vi "DataReadTxtGen.vi"(6 "VarParIndex":i32, 8 "error in":errorcluster, 9 "ScanlistIndex":i32, 10 "chemin Data":path, 11 "Chemin Header":path) -> (0 "error out":errorcluster, 1 "Y Array":dbl[](array[numeric]), 2 "X Array":dbl[](array[numeric]), 3 "Data Preview":string[][](array[string]), 4 "CurveName":string, 5 "VarPar":string)   [LabVIEW 2010]
doc: "Ce VI lit les données contenu dans le fichier de sauvegarde automatique. Ces données correspondent aux valeurs prises lors du dernier balayage. La sauvegarde automatique est effectué après chaque acquisition."
uses:
  H:/Mes documents/Programmes Labview/LabScan/LabScanV1A/Interface Class/ScanParams.ctl
  H:/Mes documents/Programmes Labview/LabScan/LabScanV1A/Interface Class/Interface.lvclass
panel:
  out "enregistrement(s)":T1={"Entête"="", "Scan list"=[], "NbCourbe"=1, "IndCourbe"=0, "NomDon"=["RTêta;", "X&Y;"], "Session "=0, "Date"="", "Time"="", "VarParams"=[], "UserName"="", "ScanTableSize"=[]} caption="ScanParams"
  out "AllData":dbl[][](array[numeric]) format="%#.16f"
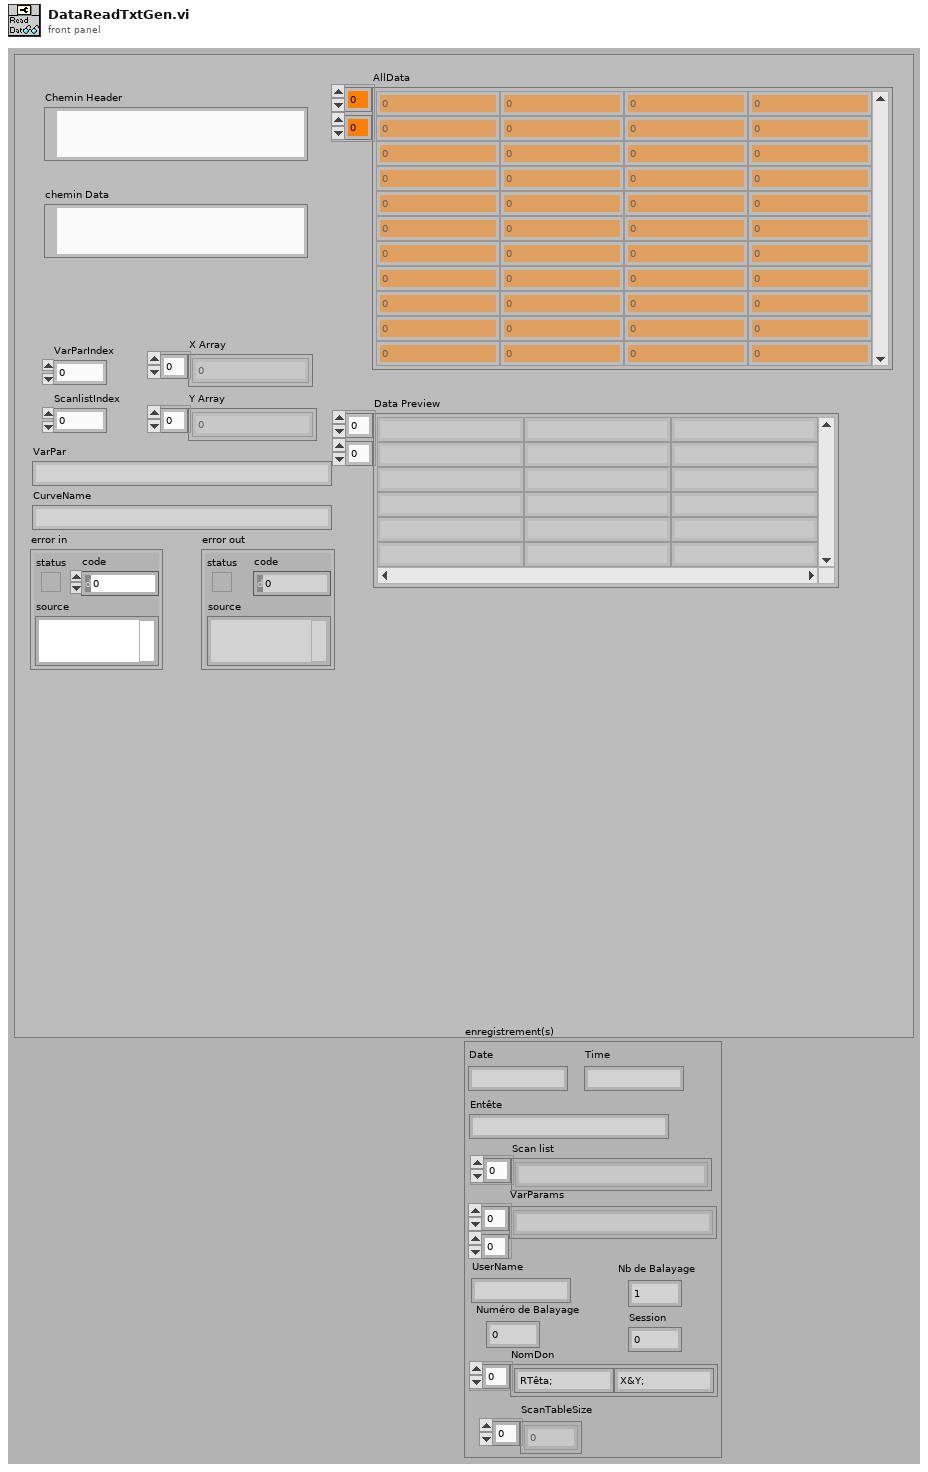
[diagram p1: front panel]
types:
  T1 = typedef "Interface.lvclass/ScanParams.ctl" = cluster{"Entête":string, "Scan list":string[], "NbCourbe":i32, "IndCourbe":i64, "NomDon":string[], "Session ":i32, "Date":string, "Time":string, "VarParams":string[][], "UserName":string, "ScanTableSize":i32[]}
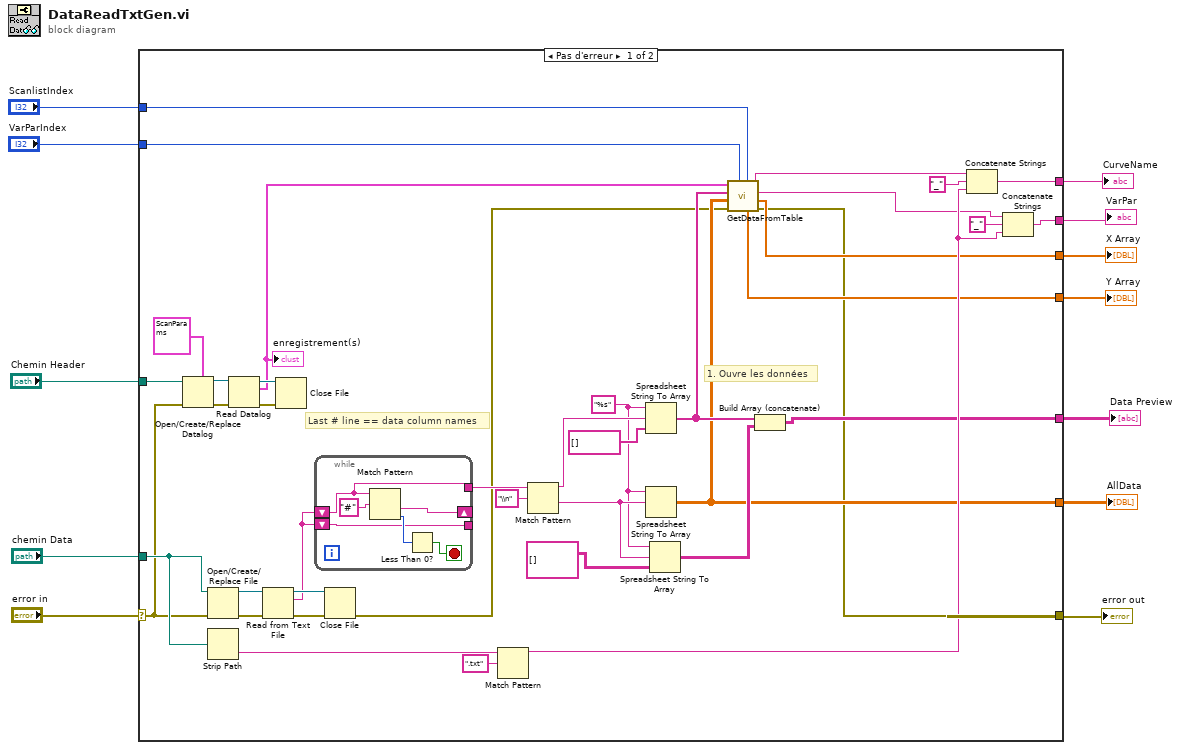
[diagram p0: block diagram]
diagram:
  n1 = case shown="Pas d'erreur" "error in" {
    selector: "error in" -> [w24 w59]
    tunnel: "chemin Data" -> [w38 _]
    tunnel: [w17 w59] -> w12
    tunnel: [w26 _] -> w9
    tunnel: [w22 _] -> w8
    tunnel: "Chemin Header" -> [w39 _]
    tunnel: "ScanlistIndex" -> [w13 _]
    tunnel: "VarParIndex" -> [w15 _]
    tunnel: [w19 _] -> w4
    tunnel: [w18 _] -> w3
    tunnel: [w32 _] -> w2
    tunnel: [w34 _] -> w1
    frame No Error {
      w28 = "%s" ("chaîne de format")
      # "Last # line == data column names"
      # "1. Ouvre les données"
      n2 = Open/Create/Replace Datalog(5:T1 {"Entête"="", "Scan list"=[], "NbCourbe"=1, "IndCourbe"=1, "NomDon"=["RTêta;", "X&Y;"], "Session "=0, "Date"="", "Time"="", "VarParams"=[], "UserName"="", "ScanTableSize"=[]} ("ScanParams"), 8:w24, 11:w39) -> (0:w43:errorcluster, 3:w42:refnum<k1>)  [unwired: 3 in, 1 out]
      n3 = Open/Create/Replace File(file path (use dialog)=w38, error in=w24) -> (refnum out=w52:refnum<file>, error out=w51:errorcluster)  [unwired: 4 in, 1 out]
      n4 = Strip Path(path=w38) -> (name=w36:string)  [unwired: 1 out]
      n5 = Read Datalog(4:w43, 7:w42) -> (0:w41:errorcluster, 2:w14:T1, 3:w40:refnum<k1>)  [unwired: 1 in]
      "enregistrement(s)" <- w14
      n6 = Read from Text File(file (use dialog)=w52, error in=w51) -> (refnum out=w49:refnum<file>, text=w45:string, error out=w50:errorcluster)  [unwired: 2 in, 1 out]
      n7 = Close File(refnum=w40, error in=w41) -> ()  [unwired: 2 out]
      n8 = while {
        shift-right: [w57] -> _
        shift-left: w45 -> [w54]
        tunnel: [w54] -> w48
        shift-left: w45 -> [w53]
        tunnel: [w53] -> _
        stop <- w55 stop-if-true
        n9 = Match Pattern(string=w54, regular expression="#" ("expression régulière")) -> (after substring=w57:string, offset past match=w56:i32)  [unwired: 1 in, 2 out]
        n10 = Less Than 0?(x=w56) -> (x < 0?=w55:bool)
      }
      n11 = Close File(refnum=w49, error in=w50) -> (error out=w16:errorcluster)  [unwired: 1 out]
      n12 = Match Pattern(string=w36, regular expression=".txt" ("expression régulière")) -> (before substring=w31:string)  [unwired: 1 in, 3 out]
      n13 = Match Pattern(string=w48, regular expression="\\n" ("expression régulière")) -> (before substring=w46:string, after substring=w30:string)  [unwired: 1 in, 2 out]
      n14 = Spreadsheet String To Array(format string=w28, spreadsheet string=w46, array type (2D Dbl)=string[] []) -> (array=w23:string[])  [unwired: 1 in]
      n15 = Spreadsheet String To Array(format string=w28, spreadsheet string=w30) -> (array=w22:dbl[][])  [unwired: 2 in]
      n16 = Spreadsheet String To Array(format string=w28, spreadsheet string=w30, array type (2D Dbl)=string[][] []) -> (array=w27:string[][])  [unwired: 1 in]
      n17 = call "GetDataFromTable.vi"("ScanlistIndex"=w13, "VarParIndex"=w15, "error in"=w16, "AllDataIn"=w22, "FilesColName"=w23, "DataRecord"=w14) -> ("error out"=w17:errorcluster, "X Array"=w18:dbl[], "VarPar"=w20:string, "CurveName"=w21:string, "Y Array"=w19:dbl[])  [unwired: 1 in]
      n18 = Build Array (concatenate)(w23, w27) -> (w26:string[][])
      n19 = Concatenate Strings(w21, "_" ("chaîne"), w31) -> (w34:string)
      n20 = Concatenate Strings(w20, "_" ("chaîne"), w31) -> (w32:string)
    }
    frame Error {
    }
  }
  "error out" <- w12
  "Data Preview" <- w9
  "AllData" <- w8
  "Y Array" <- w4
  "X Array" <- w3
  "VarPar" <- w2
  "CurveName" <- w1
